vi "FTW-TestExecutive-Core_Pause.vi"(0 "FTW-TestExecutive-Core In":refnum<class "FTW-TestExecutive-Core.lvclass">, 11 "error in":errorcluster) -> (4 "FTW-TestExecutive-Core Out":refnum<class "FTW-TestExecutive-Core.lvclass">, 15 "error out":errorcluster)   [LabVIEW 2015, in "FTW-TestExecutive-Core.lvclass"]
uses:
  FTW-TestExecutive-Core.lvclass
  FTW-TestExecutive-Core.lvclass/FTW-TestExecutive-Core.ctl
  FTW-TestExecutive-Core_State.ctl
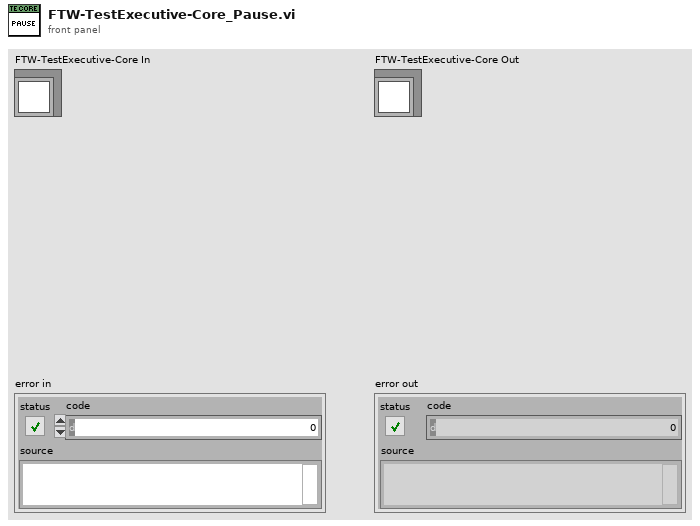
[diagram p1: front panel]
types:
  T1 = typedef "FTW-TestExecutive-Core.lvclass/FTW-TestExecutive-Core_State.ctl" = enum8{"Unloaded", "Loaded", "Executing", "Paused"}
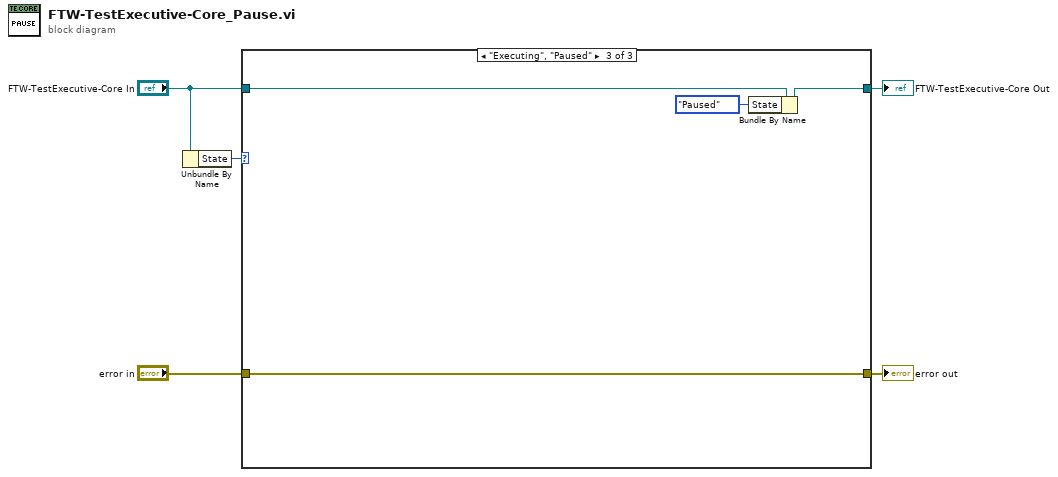
[diagram p0: block diagram]
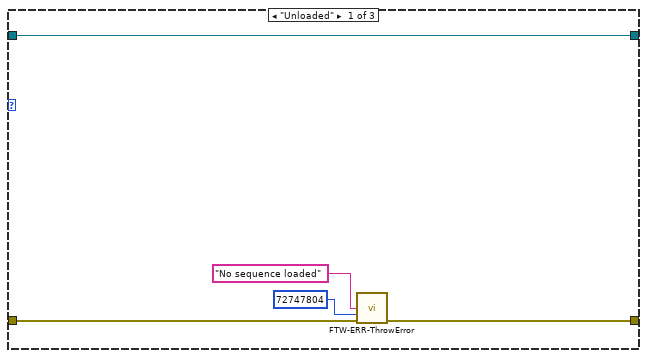
[diagram p2: hidden frame]
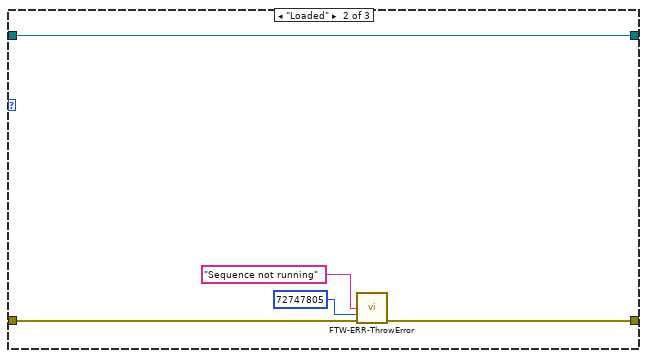
[diagram p3: hidden frame]
diagram:
  n1 = Unbundle By Name("FTW-TestExecutive-Core In") -> ("State"=w3:T1)
  n2 = case shown="\"Executing\", \"Paused\"" w3 {
    tunnel: [w10 w15 w17] -> w5
    tunnel: "FTW-TestExecutive-Core In" -> [w10 w15 w19]
    tunnel: [w8 w13 w18] -> w2
    tunnel: "error in" -> [w9 w14 w18]
    frame "Unloaded" {
      n3 = call "FTW-ERR-ThrowError.vi"("Error Message"="No sequence loaded", "Error Code"=72747804, "error in"=w9) -> ("error out"=w8:errorcluster)  [unwired: 12 in]
    }
    frame "Loaded" {
      n4 = call "FTW-ERR-ThrowError.vi"("Error Message"="Sequence not running", "Error Code"=72747805, "error in"=w14) -> ("error out"=w13:errorcluster)  [unwired: 12 in]
    }
    frame "Executing", "Paused" {
      n5 = Bundle By Name(cluster=w19, "State"=FTW-TestExecutive-Core_State."Paused") -> (w17:refnum<class "FTW-TestExecutive-Core.lvclass">)
    }
  }
  "FTW-TestExecutive-Core Out" <- w5
  "error out" <- w2
